vi "Query Arb Waveform Capabilities 64 [ARB64] Core.vi"(8 "error in (no error)":errorcluster, 11 "IVI_Fgen in":refnum<class "IVI_Fgen.lvclass">) -> (0 "error out":errorcluster, 1 "waveform quantum":i32, 2 "max number of waveforms":i32, 3 "IVI_Fgen out":refnum<class "IVI_Fgen.lvclass">, 4 "max waveform size":i64, 6 "min waveform size":i64)   [LabVIEW 2013, in "IVI_Fgen.lvlib" / "IVI_Fgen.lvclass"]
doc: "This VI returns the properties of the function generator that are related to creating arbitrary waveforms. These properties are the maximum number of waveforms, waveform quantum, minimum waveform size, and maximum waveform size.\n\nThis VI is a 64-bit version of IviFgen Query Arb Waveform Capabilities [ARB] VI.\n\nNote:\n\n(1) This VI is part of the IviFgenArbWfmSize64 [ARB64] extension group."
uses:
  IVI_Fgen.lvclass
  IVI_Fgen.lvclass/IVI_Fgen.ctl
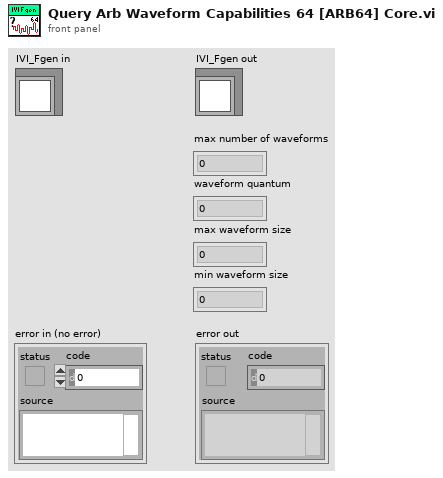
[diagram p1: front panel]
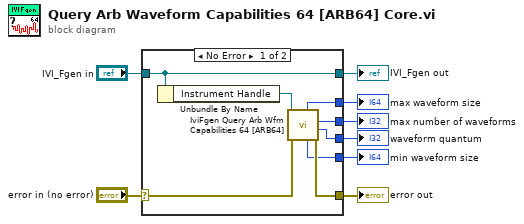
[diagram p0: block diagram]
diagram:
  n1 = case shown="No Error" "error in (no error)" {
    selector: "error in (no error)" -> [w14 w18]
    tunnel: [w13 w18] -> w7
    tunnel: [w16 w17] -> w5
    tunnel: "IVI_Fgen in" -> [w16 w17]
    tunnel: [w12 _] -> w4
    tunnel: [w11 _] -> w3
    tunnel: [w9 _] -> w2
    tunnel: [w10 _] -> w1
    frame No Error {
      n2 = Unbundle By Name(w16) -> ("Instrument Handle"=w15:refnum<k15>)
      n3 = call <vilib>:"IviFgen Query Arb Wfm Capabilities 64 [ARB64].vi"("error in (no error)"=w14, "instrument handle"=w15) -> ("error out"=w13:errorcluster, "Waveform Quantum"=w11:i32, "Maximum Number of Waveforms"=w12:i32, "Minimum Waveform Size"=w10:i64, "Maximum Waveform Size"=w9:i64)  [unwired: 4 in, 1 out]
    }
    frame Error {
    }
  }
  "error out" <- w7
  "IVI_Fgen out" <- w5
  "max number of waveforms" <- w4
  "waveform quantum" <- w3
  "max waveform size" <- w2
  "min waveform size" <- w1
